vi "AO_mini_shutdownEMCCD.vi"   [LabVIEW 2018]
panel:
  # "Shut down EMCCD"
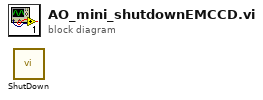
[diagram p0: block diagram]
diagram:
  n1 = call <userlib>:"ShutDown.vi"() -> ()  [unwired: 2 in, 2 out]
